vi "scan (SubVI).vi"(9 "stop":bool, 10 "dimension size 2":i32=51, 11 "dimension size":i32=51) -> (1 "enviroment":u32[][](graph), 2 "Array":u32[][](array[colorbox]), 3 "new picture":picture)   [LabVIEW 2011]
uses:
  <vilib>/Platform/TimedLoop/XDataNode/timing_clust.ctl
  <vilib>/Platform/TimedLoop/XDataNode/nitl_modes.ctl
  <vilib>/Platform/TimedLoop/XDataNode/wakeup.ctl
  <vilib>/Analysis/coordinate.llb/Angle Units.ctl
  <vilib>/Analysis/coordinate.llb/Angle Range (Degree).ctl
  <vilib>/robotics/Starter Kit/2.0/9632 Host Interface/NI_Robotics_Starter Kit Host_9632_2.0.lvclass
  <vilib>/Analysis/coordinate.llb/Wrap Angle (scalar).vi
  <vilib>/Platform/TimedLoop/XDataNode/XDataNode.xnode
  <vilib>/Platform/TimedLoop/XDataNode/XDNodeRunTimeDep.lvlib
  <vilib>/Analysis/NI_AAL_Angle.lvlib
  <vilib>/ptbypt/NI_PtbyPt.lvlib
  <vilib>/robotics/Starter Kit/Host Interface/NI_Robotics_Starter Kit Host.lvclass
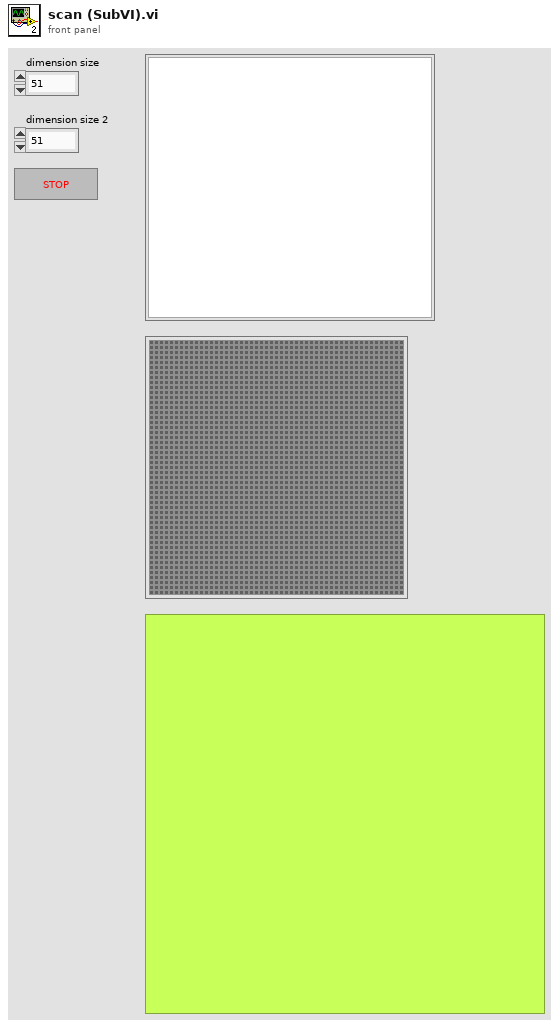
[diagram p1: front panel]
types:
  T1 = typedef "XDNodeRunTimeDep.lvlib/timing_clust.ctl" = cluster{"Expected End [f-1]":u64, "Actual End [f-1]":u64, "Finished Late? [f-1]":bool, "Expected End [i-1]":u64, "Actual End [i-1]":u64, "Finished Late? [i-1]":bool, "Expected Start [i]":u64, "Actual Start [i]":u64, "Expected Start [f]":u64, "Actual Start [f]":u64, "Source Name":string, "Structure Name":string, "Period":i64, "Deadline":i64, "Offset":i64, "Start":i64, "Priority":i32, "Timeout":i32, "Mode":T2, "Wakeup Reason":T3, "Error":errorcluster, "Source Type":string, "Secondary Source Type":string, "Global End Time":u64, "Global Start Time":u64, "Frame Duration":u64, "Iteration Duration":u64, "Assigned CPU":i32, "I/O Scan Engine Mode":u32}
  T2 = typedef "XDNodeRunTimeDep.lvlib/nitl_modes.ctl" = enum32{"No Change", "Process missed periods, maintain original phase", "Discard missed periods, maintain original phase", "Process missed periods, ignore original phase", "Discard missed periods, ignore original phase"}
  T3 = typedef "XDNodeRunTimeDep.lvlib/wakeup.ctl" = enum32{"Normal", "Aborted", "Asynchronous wakeup", "Timing source error", "Timed loop error", "Timeout"}
  T4 = typedef "NI_AAL_Angle.lvlib/Angle Units.ctl" = i32
  T5 = typedef "NI_AAL_Angle.lvlib/Angle Range (Degree).ctl" = u16
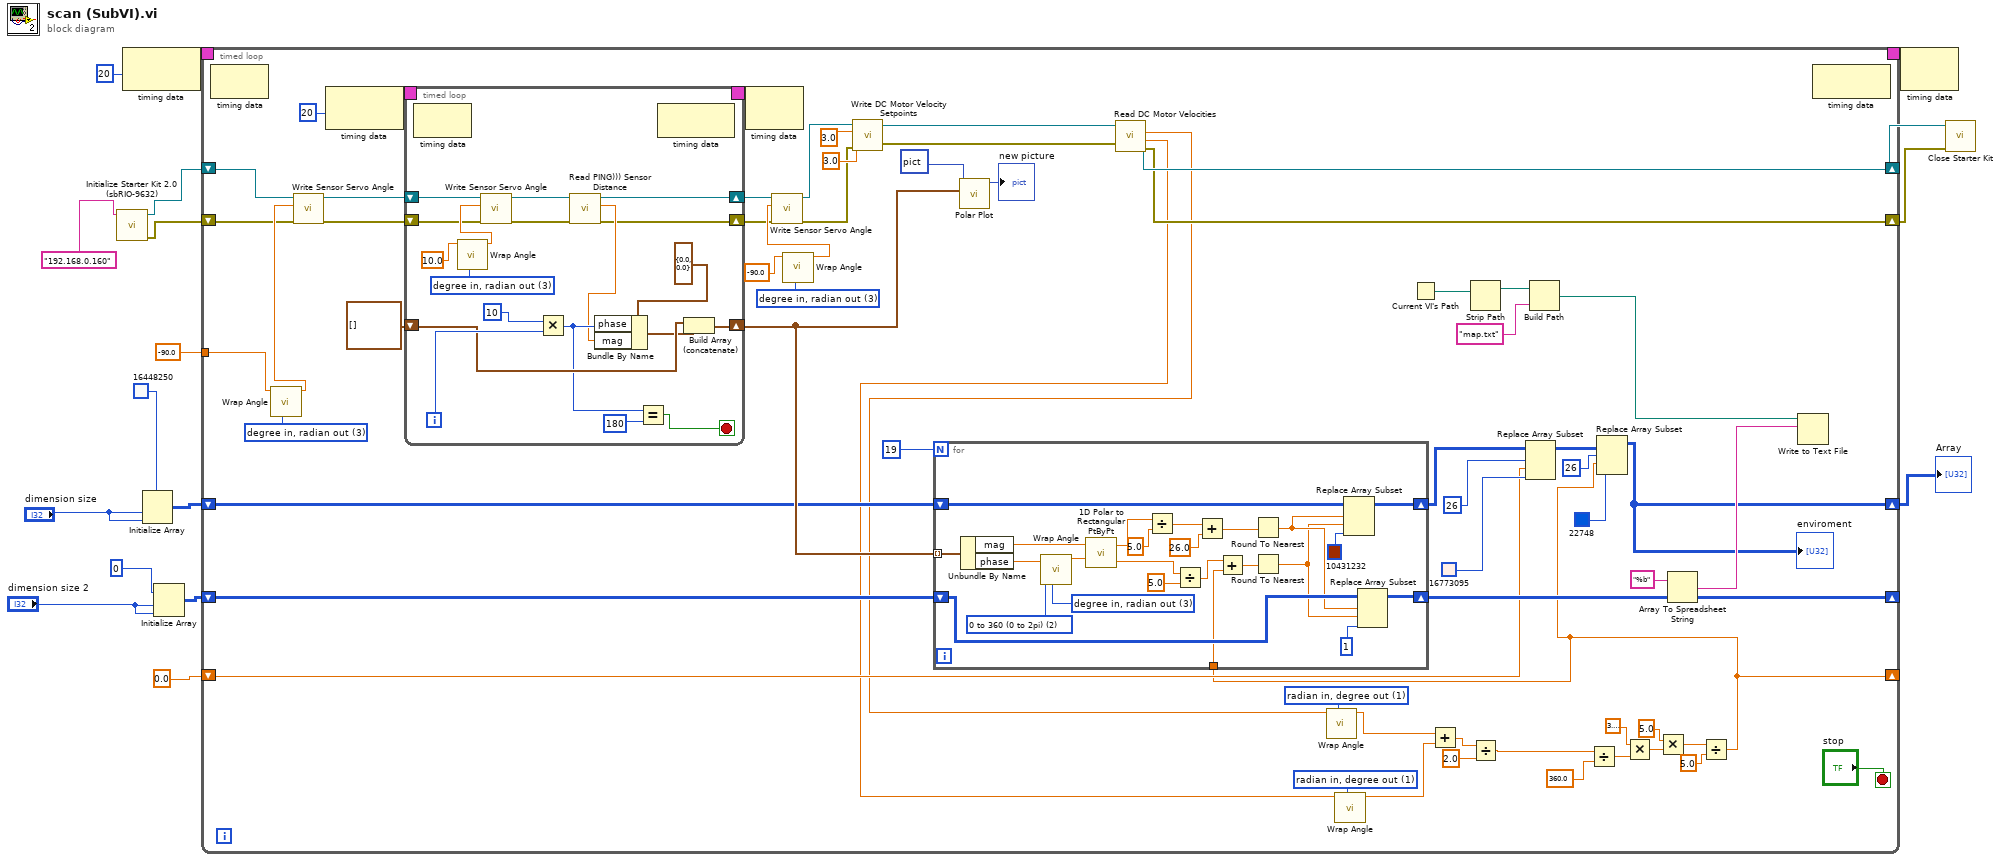
[diagram p0: block diagram]
diagram:
  n1 = call <vilib>:"Initialize Starter Kit 2.0 (sbRIO-9632).vi"("IP address (\"\")"="192.168.0.160" ("robot ID")) -> ("error out"=w5:errorcluster, "FPGA starter kit host 2.0 out"=w6:refnum<class "NI_Robotics_Starter Kit Host_9632_2.0.lvclass">)  [unwired: 9 in]
  n2 = node-c288(i64 20 ("Period")) -> (w17:T1)
  n3 = Initialize Array(u32 16448250, "dimension size", "dimension size") -> (w11:u32[][])
  n4 = Initialize Array(u32 0 ("element"), "dimension size 2", "dimension size 2") -> (w10:u32[][])
  n5 = timed-loop {
    shift-right: [w18] -> w1
    shift-left: w11 -> [w60]
    shift-right: [w62] -> _
    shift-left: w10 -> [w61]
    shift-right: [w39] -> _
    shift-left: 0.0 -> [w41]
    shift-right: [w27] -> w8
    shift-left: w6 -> [w40]
    shift-right: [w25] -> w7
    shift-left: w5 -> [w32]
    timing: w17 -> [_]
    timing-out: [_] -> w16
    tunnel: -90.0 ("angle in") -> [w19]
    stop <- "stop" stop-if-true
    w38 = T4 1 items=["radian in, radian out", "radian in, degree out", "degree in, degree out", "degree in, radian out"] ("angle units")
    w49 = T4 1 items=["radian in, radian out", "radian in, degree out", "degree in, degree out", "degree in, radian out"] ("angle units")
    w54 = T4 3 items=["radian in, radian out", "radian in, degree out", "degree in, degree out", "degree in, radian out"] ("angle units")
    w58 = T4 3 items=["radian in, radian out", "radian in, degree out", "degree in, degree out", "degree in, radian out"] ("angle units")
    n6 = node-c288 ("Output Node")() -> ()  [unwired: 1 in, 1 out]
    n7 = call-poly <vilib>:"Wrap Angle.vi"("angle units"=w54, "angle in"=w19) -> ("angle out"=w55:dbl)  [unwired: 8 in, 1 out]
    n8 = call <vilib>:"Write Sensor Servo Angle.vi"("error in (no error)"=w32, "ccw servo angle (rad)"=w55, "starter kit host in"=w40) -> ("error out"=w31:errorcluster, "starter kit host out"=w53:refnum<class "NI_Robotics_Starter Kit Host_9632_2.0.lvclass">)  [unwired: 7 in]
    n9 = node-c288(i64 20 ("Period")) -> (w22:T1)
    n10 = timed-loop {
      shift-right: [w84] -> w59
      shift-left: w53 -> [w90]
      shift-right: [w98] -> w77
      shift-left: cluster{"mag":dbl, "phase":dbl}[] [] -> [w96]
      shift-right: [w81] -> w30
      shift-left: w31 -> [w83]
      timing: w22 -> [_]
      timing-out: [_] -> w21
      i -> [w99]
      stop <- w92 stop-if-true
      w87 = T4 3 items=["radian in, radian out", "radian in, degree out", "degree in, degree out", "degree in, radian out"] ("angle units")
      n11 = node-c288() -> ()  [unwired: 1 in, 1 out]
      n12 = call-poly <vilib>:"Wrap Angle.vi"("angle units"=w87, "angle in"=10.0) -> ("angle out"=w88:dbl)  [unwired: 8 in, 1 out]
      n13 = call <vilib>:"Write Sensor Servo Angle.vi"("error in (no error)"=w83, "ccw servo angle (rad)"=w88, "starter kit host in"=w90) -> ("error out"=w82:errorcluster, "starter kit host out"=w86:refnum<class "NI_Robotics_Starter Kit Host_9632_2.0.lvclass">)  [unwired: 7 in]
      n14 = Multiply(x=10, y=w99) -> (x*y=w94:i32)
      n15 = call <vilib>:"Read PING))) Sensor Distance.vi"("error in (no error)"=w82, "starter kit host in"=w86) -> ("error out"=w81:errorcluster, "distance (m)"=w85:dbl, "starter kit host out"=w84:refnum<class "NI_Robotics_Starter Kit Host_9632_2.0.lvclass">)  [unwired: 6 in, 1 out]
      n16 = Bundle By Name(cluster=cluster{"mag":dbl, "phase":dbl} {"mag"=0.0, "phase"=0.0} ("input cluster"), "phase"=w94, "mag"=w85) -> (w95:cluster{"mag":dbl, "phase":dbl})
      n17 = Equal?(x=w94, y=180) -> (x = y?=w92:bool)
      n18 = node-c288() -> ()  [unwired: 1 in, 1 out]
      n19 = Build Array (concatenate)(w96, w95) -> (w98:cluster{"mag":dbl, "phase":dbl}[])
    }
    n20 = node-c288(w21) -> ()  [unwired: 1 out]
    n21 = call-poly <vilib>:"Wrap Angle.vi"("angle units"=w58, "angle in"=-90.0) -> ("angle out"=w56:dbl)  [unwired: 8 in, 1 out]
    n22 = call <vilib>:"Write Sensor Servo Angle.vi"("error in (no error)"=w30, "ccw servo angle (rad)"=w56, "starter kit host in"=w59) -> ("error out"=w29:errorcluster, "starter kit host out"=w50:refnum<class "NI_Robotics_Starter Kit Host_9632_2.0.lvclass">)  [unwired: 7 in]
    n23 = call <vilib>:"Write DC Motor Velocity Setpoints.vi"("error in (no error)"=w29, "right motor ccw velocity (rad/s)"=3.0, "left motor ccw velocity (rad/s)"=3.0, "starter kit host in"=w50) -> ("error out"=w26:errorcluster, "starter kit host out"=w28:refnum<class "NI_Robotics_Starter Kit Host_9632_2.0.lvclass">)  [unwired: 6 in]
    n24 = call <vilib>:"Polar Plot.vi"("data array [mag, phase (deg)]"=w77, "picture"=picture data[5B]) -> ("new picture"=→"new picture":picture)  [unwired: 9 in]
    n25 = call <vilib>:"Read DC Motor Velocities.vi"("error in (no error)"=w26, "starter kit host in"=w28) -> ("error out"=w25:errorcluster, "right motor ccw velocity (rad/s)"=w23:dbl, "left motor ccw velocity (rad/s)"=w24:dbl, "starter kit host out"=w27:refnum<class "NI_Robotics_Starter Kit Host_9632_2.0.lvclass">)  [unwired: 6 in]
    n26 = call-poly <vilib>:"Wrap Angle.vi"("angle units"=w49, "angle in"=w24) -> ("angle out"=w36:dbl)  [unwired: 8 in, 1 out]
    n27 = call-poly <vilib>:"Wrap Angle.vi"("angle units"=w38, "angle in"=w23) -> ("angle out"=w37:dbl)  [unwired: 8 in, 1 out]
    n28 = Current VI's Path() -> (path=w75:path)
    n29 = Add(x=w36, y=w37) -> (x+y=w35:dbl)
    n30 = Strip Path(path=w75) -> (stripped path=w74:path)  [unwired: 1 out]
    n31 = Divide(x=w35, y=2.0) -> (x/y=w33:dbl)
    n32 = Build Path(base path=w74, name or relative path="map.txt") -> (appended path=w72:path)
    n33 = Divide(x=w33, y=360.0) -> (x/y=w47:dbl)
    n34 = Multiply(x=3.141592653589793, y=w47) -> (x*y=w46:dbl)
    n35 = Multiply(x=5.0, y=w46) -> (x*y=w43:dbl)
    n36 = Divide(x=w43, y=5.0) -> (x/y=w39:dbl)
    n37 = for {
      N: 19 -> [_]
      tunnel: w77 -> [w131] mode=indexing
      shift-right: [w128] -> w69
      shift-left: w60 -> [w129]
      shift-right: [w115] -> w62
      shift-left: w61 -> [w114]
      tunnel: w39 -> [w108]
      w126 = T5 2 items=["none", "-180 to 180 (-pi to pi)", "0 to 360 (0 to 2pi)"] ("angle range")
      w127 = T4 3 items=["radian in, radian out", "radian in, degree out", "degree in, degree out", "degree in, radian out"] ("angle units")
      n38 = Unbundle By Name(w131) -> ("mag"=w130:dbl, "phase"=w125:dbl)
      n39 = call-poly <vilib>:"Wrap Angle.vi"("angle units"=w127, "angle range"=w126, "angle in"=w125) -> ("angle out"=w124:dbl)  [unwired: 7 in, 1 out]
      n40 = call <vilib>:"1D Polar to Rectangular PtByPt.vi"("phase"=w124, "magnitude"=w130) -> ("y"=w117:dbl, "x"=w123:dbl)
      n41 = Divide(x=w123, y=5.0) -> (x/y=w120:dbl)
      n42 = Divide(x=w117, y=5.0) -> (x/y=w110:dbl)
      n43 = Add(x=w120, y=26.0) -> (x+y=w119:dbl)
      n44 = Add(x=w110, y=w108) -> (x+y=w109:dbl)
      n45 = Round To Nearest(number=w119) -> (nearest integer value=w113:dbl)
      n46 = Round To Nearest(number=w109) -> (nearest integer value=w112:dbl)
      n47 = Replace Array Subset(array=w129, new element=u32 10431232, index (row)=w113, index (col)=w112) -> (w128:u32[][])
      n48 = Replace Array Subset(array=w114, new element=u32 1 ("new element/subarray"), index (row)=w113, index (col)=w112) -> (w115:u32[][])
    }
    n49 = Replace Array Subset(array=w69, new element=u32 16773095, index (row)=26, index (col)=w41) -> (w65:u32[][])
    n50 = Replace Array Subset(array=w65, new element=u32 22748, index (row)=26, index (col)=w39) -> (w18:u32[][])
    "enviroment" <- w18
    n51 = Array To Spreadsheet String(array=w62, 3:"%b" ("format string")) -> (spreadsheet string=w71:string)  [unwired: 1 in]
    n52 = Write to Text File(file (use dialog)=w72, text=w71) -> ()  [unwired: 2 in, 3 out]
    n53 = node-c288() -> ()  [unwired: 1 in, 1 out]
  }
  "Array" <- w1
  n54 = node-c288(w16) -> ()  [unwired: 1 out]
  n55 = call-dynamic "Close Starter Kit.vi"("error in (no error)"=w7, "starter kit host in"=w8) -> ()  [unwired: 9 in, 1 out]
